vi "Convert Joystick Button Event Data.vi"(11 "Event Data":u8[](array[numeric]) format="%.0x") -> (3 "Joystick Button Event":T1 {"State" format="%.0x"; "Which" format="%.0x"; "Type" format="%.0x"})   [LabVIEW 2015, in "LibSDL2.lvlib"]
uses:
  LibSDL2.lvlib
  Controls/Joysitck Button Event.ctl
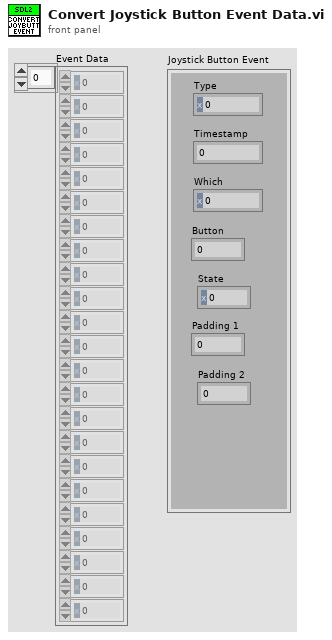
[diagram p1: front panel]
types:
  T1 = typedef "LibSDL2.lvlib/Joysitck Button Event.ctl" = cluster{"Type":u32, "Timestamp":u32, "Which":i32, "Button":u8, "State":u8, "Padding 1":u8, "Padding 2":u8}
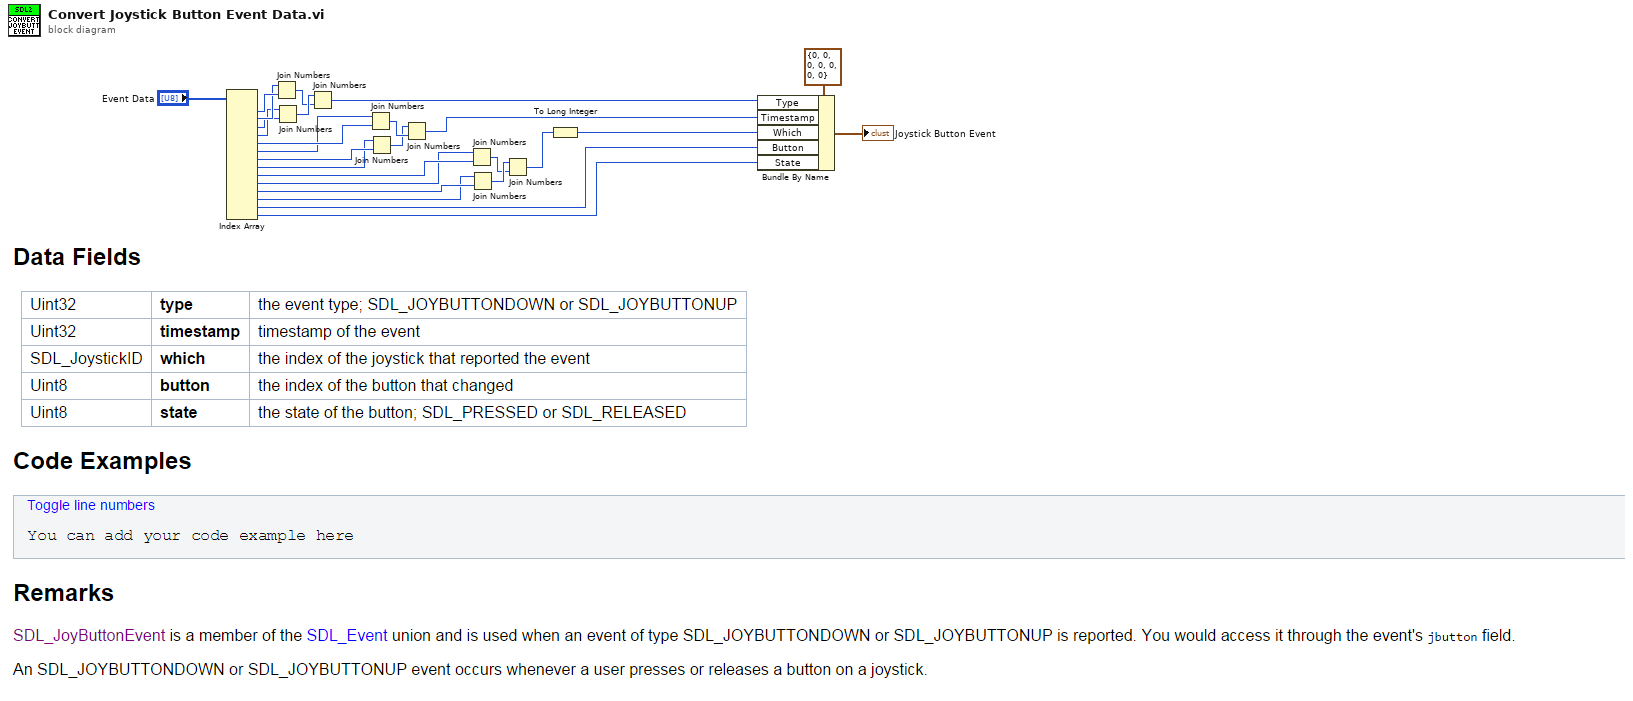
[diagram p0: block diagram]
diagram:
  n1 = Index Array(array="Event Data") -> (element #1=w25:u8, element #2=w24:u8, element #3=w22:u8, element #4=w23:u8, element #5=w16:u8, element #6=w15:u8, element #7=w14:u8, element #8=w13:u8, element #9=w9:u8, element #10=w8:u8, element #11=w7:u8, element #12=w6:u8, element #13=w5:u8, element #14=w4:u8)  [unwired: 14 in]
  n2 = Join Numbers(hi=w24, lo=w25) -> ((hi.lo)=w20:u16)
  n3 = Join Numbers(hi=w23, lo=w22) -> ((hi.lo)=w21:u16)
  n4 = Join Numbers(hi=w21, lo=w20) -> ((hi.lo)=w19:u32)
  n5 = Join Numbers(hi=w15, lo=w16) -> ((hi.lo)=w18:u16)
  n6 = Join Numbers(hi=w13, lo=w14) -> ((hi.lo)=w17:u16)
  n7 = Join Numbers(hi=w17, lo=w18) -> ((hi.lo)=w12:u32)
  n8 = Join Numbers(hi=w8, lo=w9) -> ((hi.lo)=w10:u16)
  n9 = Join Numbers(hi=w6, lo=w7) -> ((hi.lo)=w11:u16)
  n10 = Join Numbers(hi=w11, lo=w10) -> ((hi.lo)=w3:u32)
  n11 = To Long Integer(number=w3) -> (32bit integer=w2:i32)
  n12 = Bundle By Name(cluster=T1 {"Type"=0, "Timestamp"=0, "Which"=0, "Button"=0, "State"=0, "Padding 1"=0, "Padding 2"=0} ("Joystick Button Event"), "Type"=w19, "Timestamp"=w12, "Which"=w2, "Button"=w5, "State"=w4) -> (→"Joystick Button Event":T1)
